vi "SearchSdlDllInGObjects.vi"(8 "error in (no error)":errorcluster, 11 "Diagram GObjects":refnum<vi>[](array[refnum])) -> (0 "error out":errorcluster, 2 "SDL DLLs":refnum<vi>[](array[refnum]))   [LabVIEW 2024, in "CustomActions.lvlib"]
uses:
  CustomActions.lvlib
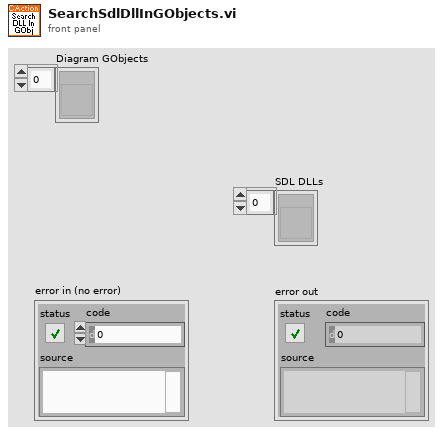
[diagram p1: front panel]
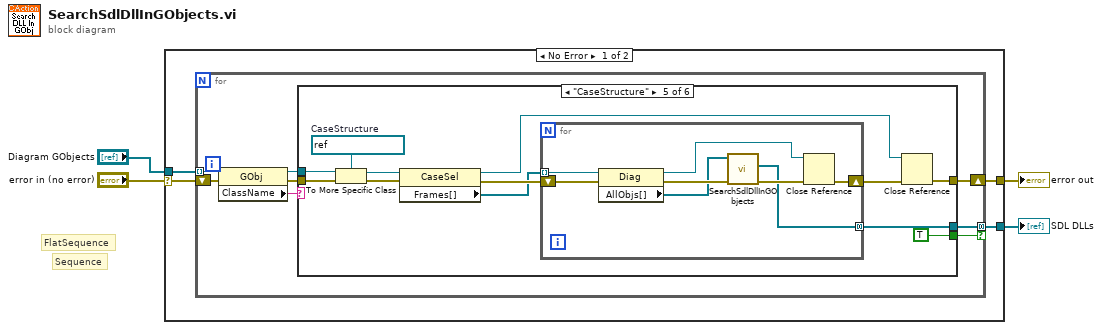
[diagram p0: block diagram]
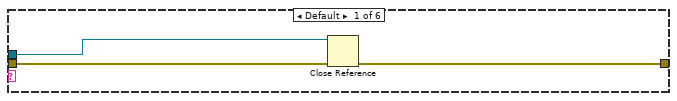
[diagram p2: hidden frame]
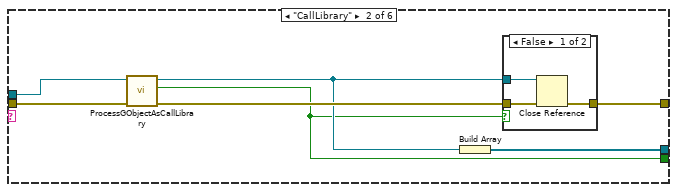
[diagram p3: hidden frame]
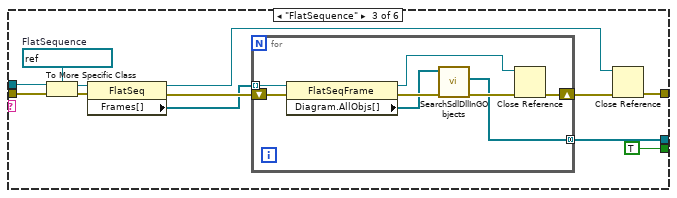
[diagram p5: hidden frame]
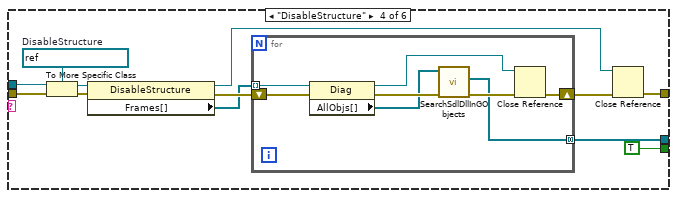
[diagram p6: hidden frame]
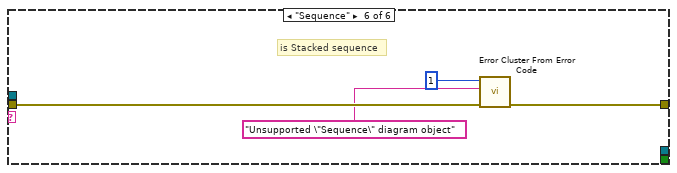
[diagram p7: hidden frame]
diagram:
  # "Sequence"
  # "FlatSequence"
  n1 = case shown="No Error" "error in (no error)" {
    selector: "error in (no error)" -> [w5 w95]
    tunnel: [w8 _] -> w4
    tunnel: [w7 w95] -> w3
    tunnel: "Diagram GObjects" -> [w6 _]
    frame No Error {
      n2 = for {
        tunnel: w6 -> [w15] mode=indexing
        shift-right: [w13] -> w7
        shift-left: w5 -> [w16]
        tunnel: [w10] -> w8 mode=concatenating if=w11
        n3 = property class="GObj"(reference=w15, error in=w16) -> (reference out=w12:refnum<vi>, error out=w14:errorcluster, "ClassName"=w9:string)
        n4 = case shown="\"CaseStructure\"" w9 {
          tunnel: w14 -> [w19 w25 w42 w62 w82 w94]
          tunnel: [w18 w26 w34 w54 w74 w93] -> w13
          tunnel: w12 -> [w17 w24 w41 w61 w81 _]
          tunnel: [_ w21 TRUE ("Is SDL?") TRUE ("Is SDL?") TRUE ("Is SDL?") _] -> w11
          tunnel: [_ w20 w32 w52 w72 _] -> w10
          frame Default {
            n5 = Close Reference(reference=w17, error in (no error)=w19) -> (error out=w18:errorcluster)
          }
          frame "CallLibrary" {
            n6 = call "ProcessGObjectAsCallLibrary.vi"("error in"=w25, "GObject Ref"=w24) -> ("error out"=w23:errorcluster, "Is SDL?"=w21:bool, "GObject Ref As Call Library"=w22:refnum<vi>)  [unwired: 7 in]
            n7 = Build Array(w22) -> (w20:refnum<vi>[])
            n8 = case shown="False" w21 {
              tunnel: w23 -> [w29 w30]
              tunnel: [w28 w30] -> w26
              tunnel: w22 -> [w27 _]
              frame False {
                n9 = Close Reference(reference=w27, error in (no error)=w29) -> (error out=w28:errorcluster)
              }
              frame True {
              }
            }
          }
          frame "FlatSequence" {
            w40 = refnum<vi> refnum  # FlatSequence
            n10 = To More Specific Class(target class=w40, reference=w41, error in=w42) -> (specific class reference=w39:refnum<vi>, error out=w38:errorcluster)
            n11 = property class="FlatSeq"(reference=w39, error in=w38) -> (reference out=w33:refnum<vi>, error out=w37:errorcluster, "Frames[]"=w36:refnum<vi>[])
            n12 = for {
              shift-right: [w44] -> w35
              shift-left: w37 -> [w50]
              tunnel: w36 -> [w49] mode=indexing
              tunnel: [w45] -> w32 mode=concatenating
              n13 = property class="FlatSeqFrame"(reference=w49, error in=w50) -> (reference out=w43:refnum<vi>, error out=w48:errorcluster, "Diagram.AllObjs[]"=w47:refnum<vi>[])
              n14 = call "SearchSdlDllInGObjects.vi"("error in (no error)"=w48, "Diagram GObjects"=w47) -> ("error out"=w46:errorcluster, "SDL DLLs"=w45:refnum<vi>[])  [unwired: 8 in]
              n15 = Close Reference(reference=w43, error in (no error)=w46) -> (error out=w44:errorcluster)
            }
            n16 = Close Reference(reference=w33, error in (no error)=w35) -> (error out=w34:errorcluster)
          }
          frame "DisableStructure" {
            w60 = refnum<vi> refnum  # DisableStructure
            n17 = To More Specific Class(target class=w60, reference=w61, error in=w62) -> (specific class reference=w59:refnum<vi>, error out=w58:errorcluster)
            n18 = property class="DisableStructure"(reference=w59, error in=w58) -> (reference out=w53:refnum<vi>, error out=w57:errorcluster, "Frames[]"=w56:refnum<vi>[])
            n19 = for {
              shift-right: [w64] -> w55
              shift-left: w57 -> [w70]
              tunnel: w56 -> [w69] mode=indexing
              tunnel: [w65] -> w52 mode=concatenating
              n20 = property class="Diag"(reference=w69, error in=w70) -> (reference out=w63:refnum<vi>, error out=w68:errorcluster, "AllObjs[]"=w67:refnum<vi>[])
              n21 = call "SearchSdlDllInGObjects.vi"("error in (no error)"=w68, "Diagram GObjects"=w67) -> ("error out"=w66:errorcluster, "SDL DLLs"=w65:refnum<vi>[])  [unwired: 8 in]
              n22 = Close Reference(reference=w63, error in (no error)=w66) -> (error out=w64:errorcluster)
            }
            n23 = Close Reference(reference=w53, error in (no error)=w55) -> (error out=w54:errorcluster)
          }
          frame "CaseStructure" {
            w80 = refnum<vi> refnum  # CaseStructure
            n24 = To More Specific Class(target class=w80, reference=w81, error in=w82) -> (specific class reference=w79:refnum<vi>, error out=w78:errorcluster)
            n25 = property class="CaseSel"(reference=w79, error in=w78) -> (reference out=w73:refnum<vi>, error out=w77:errorcluster, "Frames[]"=w76:refnum<vi>[])
            n26 = for {
              shift-right: [w84] -> w75
              shift-left: w77 -> [w90]
              tunnel: w76 -> [w89] mode=indexing
              tunnel: [w85] -> w72 mode=concatenating
              n27 = property class="Diag"(reference=w89, error in=w90) -> (reference out=w83:refnum<vi>, error out=w88:errorcluster, "AllObjs[]"=w87:refnum<vi>[])
              n28 = call "SearchSdlDllInGObjects.vi"("error in (no error)"=w88, "Diagram GObjects"=w87) -> ("error out"=w86:errorcluster, "SDL DLLs"=w85:refnum<vi>[])  [unwired: 8 in]
              n29 = Close Reference(reference=w83, error in (no error)=w86) -> (error out=w84:errorcluster)
            }
            n30 = Close Reference(reference=w73, error in (no error)=w75) -> (error out=w74:errorcluster)
          }
          frame "Sequence" {
            # "is Stacked sequence"
            n31 = call <vilib>:"Error Cluster From Error Code.vi"("error in (no error)"=w94, "error message (\"\")"="Unsupported \"Sequence\" diagram object" ("error message (\"\")"), "error code (0)"=1) -> ("error out"=w93:errorcluster)  [unwired: 6 in]
          }
        }
      }
    }
    frame Error {
    }
  }
  "SDL DLLs" <- w4
  "error out" <- w3
